vi "prueba_casos.vi"() -> ()   [LabVIEW 2019]
panel:
  in  "Go2":bool
  in  "Go1":bool
  out "String":string
  out "Tiempo":dbl
  out "Vel Final":dbl
  out "Vel Inicial":dbl
  out "Pos final":dbl
  in  "MOTORES INDEPENDIENTES":bool
  in  "Posición final Motor 2":dbl
  in  "Velocidad inicial Motor 2":dbl
  in  "Velocidad final Motor 2":dbl
  in  "Aceleración inicial Motor 2":dbl
  in  "Aceleración final Motor 2":dbl
  in  "Tiempo 2":dbl
  in  "Posición final motor 1":dbl
  in  "Velocidad inicial Motor 1":dbl
  in  "Velocidad final Motor 1":dbl
  in  "Aceleración inicial Motor 1":dbl
  in  "Aceleración final Motor 1":dbl
  in  "Tiempo 1":dbl
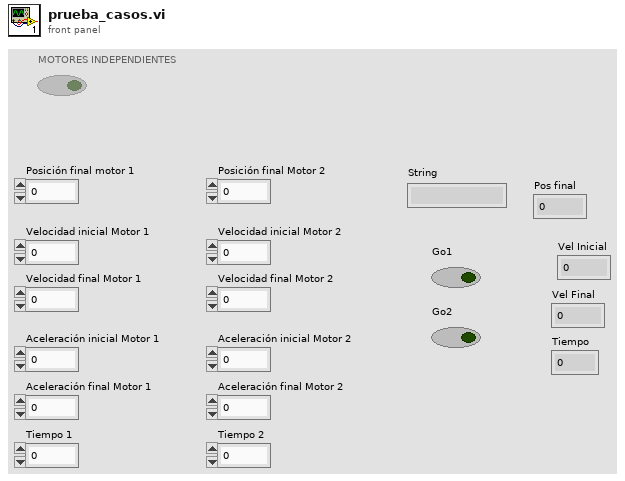
[diagram p1: front panel]
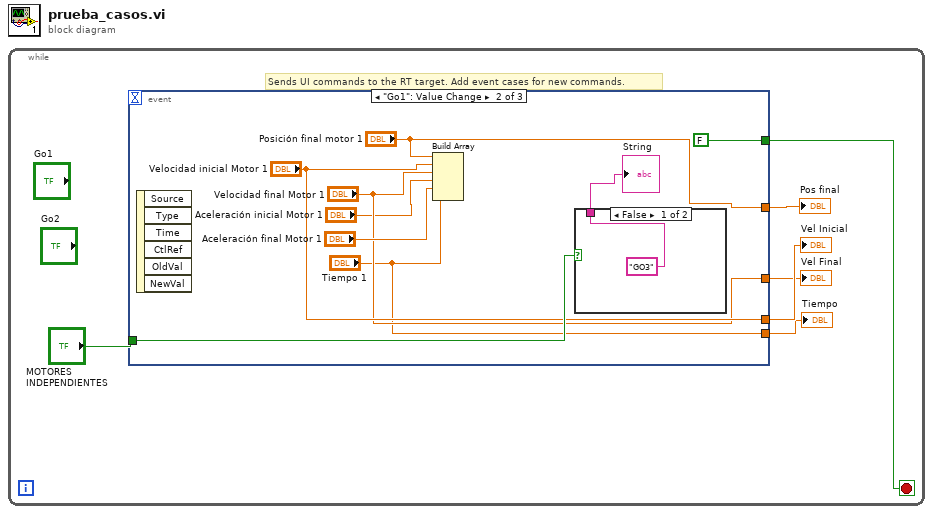
[diagram p0: block diagram]
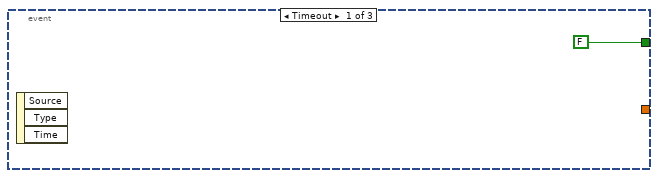
[diagram p2: hidden frame]
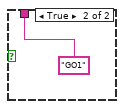
[diagram p3: hidden frame]
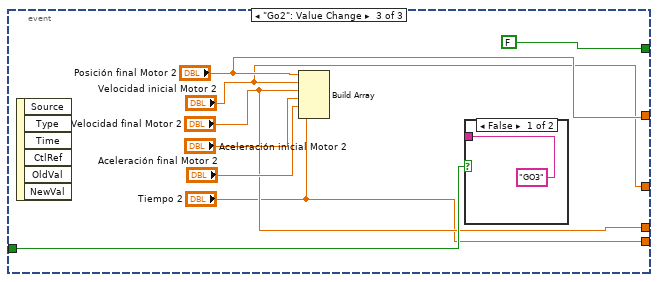
[diagram p4: hidden frame]
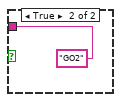
[diagram p5: hidden frame]
diagram:
  n1 = while {
    stop <- w1 stop-if-true
    # "Sends UI commands to the RT target. Add event cases for new commands."
    n2 = event shown="[1] \"Go1\": Value Change" {
      selector: _ -> [_ _ _]
      dyn-events: _ -> [_ _ _]
      timeout: _ -> [_ _ _]
      tunnel: [FALSE ("Stop UI and RT") FALSE ("Stop UI and RT") FALSE ("Stop UI and RT")] -> w1
      tunnel: "MOTORES INDEPENDIENTES" -> [_ w14 w23]
      tunnel: [_ "Posición final motor 1" "Posición final Motor 2"] -> w5
      tunnel: [_ "Velocidad inicial Motor 1" "Velocidad final Motor 2"] -> w4
      tunnel: [_ "Velocidad final Motor 1" "Velocidad inicial Motor 2"] -> w3
      tunnel: [_ "Tiempo 1" "Tiempo 2"] -> w2
      event Timeout {
        n3 = event-data() -> ()  [unwired: 1 in, 3 out]
      }
      event "Go1": Value Change {
        n4 = event-data() -> ()  [unwired: 1 in, 6 out]
        n5 = Build Array("Posición final motor 1", "Velocidad inicial Motor 1", "Velocidad final Motor 1", "Aceleración inicial Motor 1", "Aceleración final Motor 1", "Tiempo 1") -> ()  [unwired: 1 out]
        n6 = case shown="False" w14 {
          tunnel: ["GO3" ("writer name") "GO1" ("writer name")] -> w8
          frame False {
          }
          frame True {
          }
        }
        "String" <- w8
      }
      event "Go2": Value Change {
        n7 = event-data() -> ()  [unwired: 1 in, 6 out]
        n8 = Build Array("Posición final Motor 2", "Velocidad inicial Motor 2", "Velocidad final Motor 2", "Aceleración inicial Motor 2", "Aceleración final Motor 2", "Tiempo 2") -> ()  [unwired: 1 out]
        n9 = case shown="False" w23 {
          tunnel: ["GO3" ("writer name") "GO2" ("writer name")] -> _
          frame False {
          }
          frame True {
          }
        }
      }
    }
    "Pos final" <- w5
    "Vel Inicial" <- w4
    "Vel Final" <- w3
    "Tiempo" <- w2
  }
